vi "Proportional area crop.vi"(4 "multiline":u16, 6 "Cropped to area pixels":u32=1048576, 7 "keep aspect ratio":bool=TRUE, 8 "Y grids":u8=1, 9 "Y resolution":u32, 10 "X grids":u8=1, 11 "X resolution":u32) -> (0 "Y length":u32, 1 "Y index":u32[](array[numeric]), 2 "X length":u32, 3 "X index":u32[](array[numeric]), 5 "Grid settings":T1)   [LabVIEW 2018]
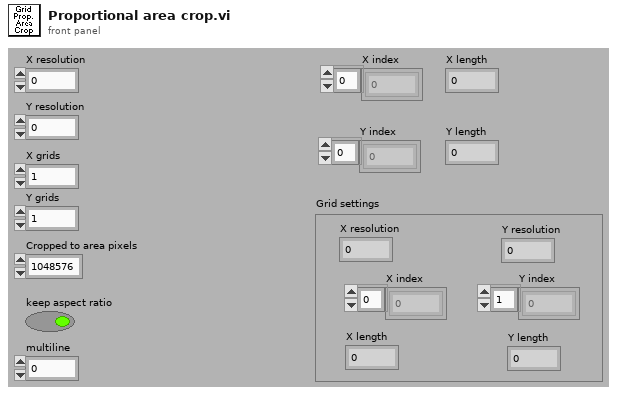
[diagram p1: front panel]
types:
  T1 = cluster{"X resolution":u32, "Y resolution":u32, "X index":u32[], "Y index":u32[], "X length":u32, "Y length":u32}
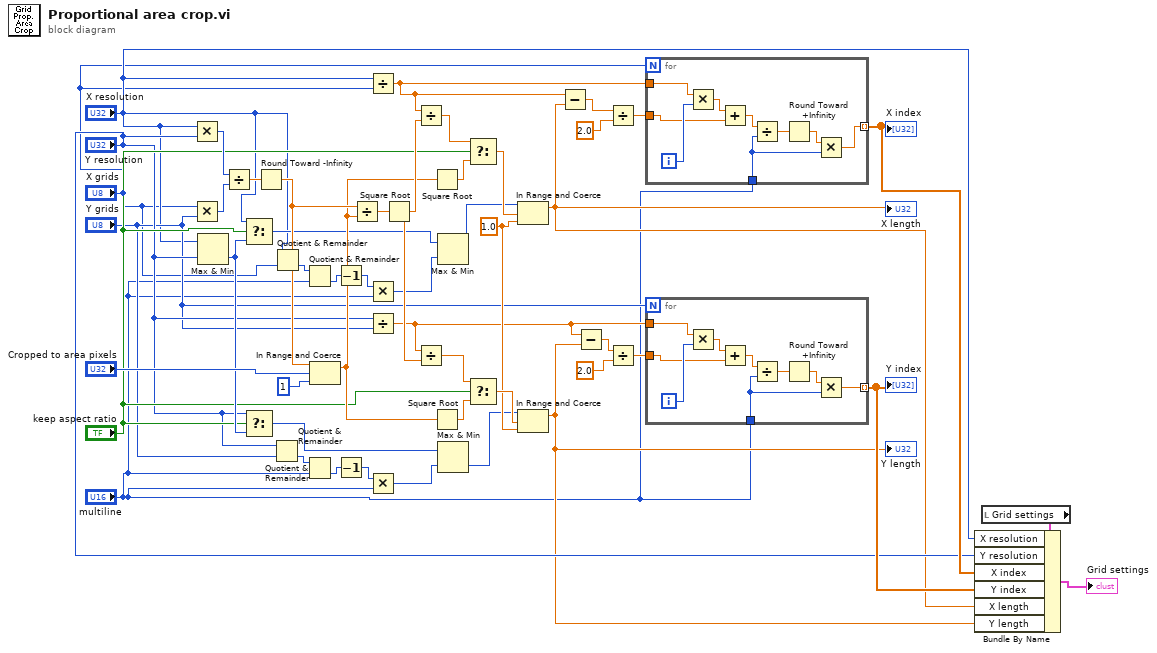
[diagram p0: block diagram]
diagram:
  w23 = 1.0 ("lower limit")
  n1 = Multiply(x="X resolution", y="Y resolution") -> (x*y=w39:u32)
  n2 = Multiply(x="X grids", y="Y grids") -> (x*y=w41:u8)
  n3 = Max & Min(x="X resolution", y="Y resolution") -> (min(x,y)=w22:u32)  [unwired: 1 out]
  n4 = Divide(x=w39, y=w41) -> (x/y=w40:dbl)
  n5 = Select(t="X resolution", s="keep aspect ratio", f=w22) -> (s? t:f=w16:u32)
  n6 = Select(t="Y resolution", s="keep aspect ratio", f=w22) -> (s? t:f=w20:u32)
  n7 = Round Toward -Infinity(1:w40) -> (0:w36:dbl)
  n8 = Quotient & Remainder(x="Y resolution", y="Y grids") -> (floor(x/y)=w7:u32)  [unwired: 1 out]
  n9 = Quotient & Remainder(x="X resolution", y="X grids") -> (floor(x/y)=w10:u32)  [unwired: 1 out]
  n10 = Quotient & Remainder(x=w10, y="multiline") -> (floor(x/y)=w9:u32)  [unwired: 1 out]
  n11 = Quotient & Remainder(x=w7, y="multiline") -> (floor(x/y)=w6:u32)  [unwired: 1 out]
  n12 = In Range and Coerce(upper limit=w36, x="Cropped to area pixels", lower limit=u32 1) -> (coerced(x)=w30:dbl)  [unwired: 1 out]
  n13 = Decrement(x=w9) -> (x-1=w1:u32)
  n14 = Decrement(x=w6) -> (x-1=w3:u32)
  n15 = Divide(x=w36, y=w30) -> (x/y=w45:dbl)
  n16 = Divide(x="X resolution", y="X grids") -> (x/y=w35:dbl)
  n17 = Multiply(x=w1, y="multiline") -> (x*y=w8:u32)
  n18 = Divide(x="Y resolution", y="Y grids") -> (x/y=w4:dbl)
  n19 = Multiply(x=w3, y="multiline") -> (x*y=w5:u32)
  n20 = Square Root(x=w45) -> (sqrt(x)=w44:dbl)
  n21 = Divide(x=w35, y=w44) -> (x/y=w34:dbl)
  n22 = Divide(x=w4, y=w44) -> (x/y=w31:dbl)
  n23 = Square Root(x=w30) -> (sqrt(x)=w33:dbl)
  n24 = Square Root(x=w30) -> (sqrt(x)=w32:dbl)
  n25 = Max & Min(x=w16, y=w8) -> (min(x,y)=w15:u32)  [unwired: 1 out]
  n26 = Max & Min(x=w20, y=w5) -> (min(x,y)=w19:u32)  [unwired: 1 out]
  n27 = Select(t=w34, s="keep aspect ratio", f=w33) -> (s? t:f=w25:dbl)
  n28 = Select(t=w31, s="keep aspect ratio", f=w32) -> (s? t:f=w24:dbl)
  n29 = In Range and Coerce(upper limit=w15, x=w25, lower limit=w23) -> (coerced(x)=w11:dbl)  [unwired: 1 out]
  "X length" <- w11
  n30 = In Range and Coerce(upper limit=w19, x=w24, lower limit=w23) -> (coerced(x)=w12:dbl)  [unwired: 1 out]
  "Y length" <- w12
  n31 = Subtract(x=w35, y=w11) -> (x-y=w46:dbl)
  n32 = Subtract(x=w4, y=w12) -> (x-y=w49:dbl)
  n33 = Divide(x=w46, y=2.0) -> (x/y=w38:dbl)
  n34 = Divide(x=w49, y=2.0) -> (x/y=w37:dbl)
  n35 = for {
    N: "X grids" -> [_]
    tunnel: w38 -> [w55]
    tunnel: w35 -> [w57]
    tunnel: [w51] -> w26 mode=indexing
    tunnel: "multiline" -> [w50]
    i -> [w58]
    n36 = Multiply(x=w57, y=w58) -> (x*y=w56:dbl)
    n37 = Add(x=w56, y=w55) -> (x+y=w52:dbl)
    n38 = Divide(x=w52, y=w50) -> (x/y=w54:dbl)
    n39 = Round Toward +Infinity(x=w54) -> (ceil(x): smallest int >= x=w53:dbl)
    n40 = Multiply(x=w53, y=w50) -> (x*y=w51:dbl)
  }
  "X index" <- w26
  n41 = for {
    N: "Y grids" -> [_]
    tunnel: w37 -> [w64]
    tunnel: w4 -> [w66]
    tunnel: [w60] -> w27 mode=indexing
    tunnel: "multiline" -> [w59]
    i -> [w67]
    n42 = Multiply(x=w66, y=w67) -> (x*y=w65:dbl)
    n43 = Add(x=w65, y=w64) -> (x+y=w61:dbl)
    n44 = Divide(x=w61, y=w59) -> (x/y=w62:dbl)
    n45 = Round Toward +Infinity(x=w62) -> (ceil(x): smallest int >= x=w63:dbl)
    n46 = Multiply(x=w63, y=w59) -> (x*y=w60:dbl)
  }
  "Y index" <- w27
  n47 = local read "Grid settings"() -> (w29:T1)
  n48 = Bundle By Name(cluster=w29, "X resolution"="X resolution", "Y resolution"="Y resolution", "X index"=w26, "Y index"=w27, "X length"=w11, "Y length"=w12) -> (→"Grid settings":T1)
